vi "SUB_VI_lettura_messaggio.vi"(8 "Errore ingresso":errorcluster, 11 "TCP Network Connection in":refnum<k5>) -> (0 "Errore uscita":errorcluster, 1 "Byte da leggere":i32, 2 "Messaggio ricevuto":string, 3 "TCP Network Connection out":refnum<k5>)   [LabVIEW 2023]
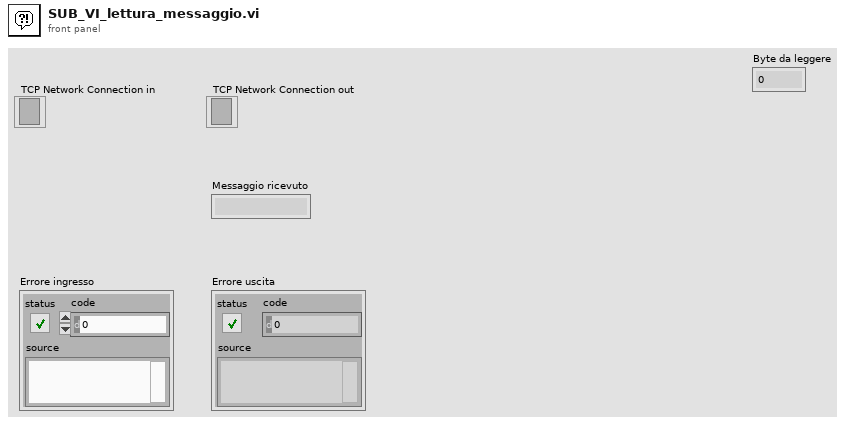
[diagram p1: front panel]
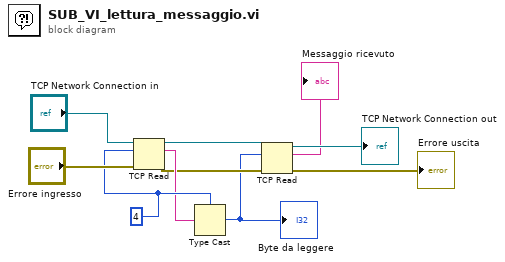
[diagram p0: block diagram]
diagram:
  w8 = 4 ("bytes to read")
  n1 = TCP Read(connection ID="TCP Network Connection in", bytes to read=w8, error in (no error)="Errore ingresso") -> (connection ID out=w2:refnum<k5>, data out=w4:string, error out=w3:errorcluster)  [unwired: 2 in]
  n2 = Type Cast(type=w8, x=w4) -> (*(type *) &x=w1:i32)
  "Byte da leggere" <- w1
  n3 = TCP Read(connection ID=w2, bytes to read=w1, error in (no error)=w3) -> (connection ID out=→"TCP Network Connection out":refnum<k5>, data out=→"Messaggio ricevuto":string, error out=→"Errore uscita":errorcluster)  [unwired: 2 in]
